vi "Photobleach.vi"(8 "error in (no error)":errorcluster, 10 "Custom Length":dbl=-9999.0, 11 "Stage Controller in":refnum<class "Stage Controller.lvclass">) -> (0 "error out":errorcluster, 3 "Stage Controller out":refnum<class "Stage Controller.lvclass">)   [LabVIEW 2018, in "Stage Controller.lvlib" / "Stage Controller.lvclass"]
uses:
  Stage Controller.lvclass
  Stage Controller.lvclass/Stage Controller.ctl
  <instrlib>/ASI TG-1000/Public/Utility/Axis Name.ctl
  Resources/GLOBAL/GLOBAL Time-critical.vi
  Ti2/ti2lv/ti2lv.lvlib
  <instrlib>/ASI TG-1000/ASI TG-1000.lvlib
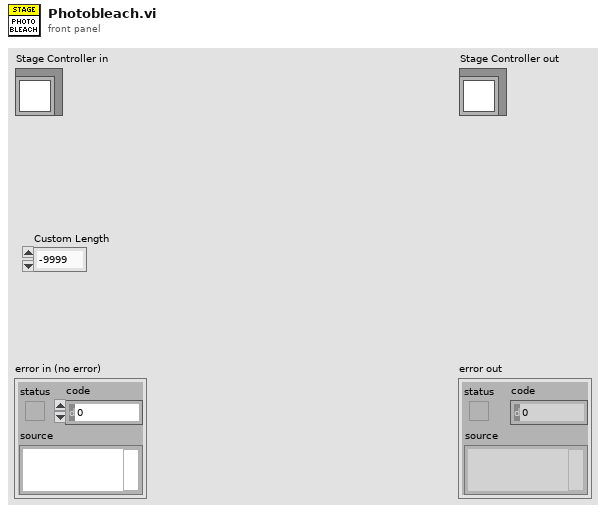
[diagram p1: front panel]
types:
  T1 = enum16{"Disabled", "ESP301", "Ti2", "Ludl", "ASI"}
  T2 = typedef "ASI TG-1000.lvlib/Axis Name.ctl" = enum8{"undefined", "A", "B", "C", "D", "E", "F", "G", "H", "I", "J", "K", "L", "M", "N", "O", "P", "Q", "R", "S", "T", "U", "V", "W", "X", "Y", "Z"}
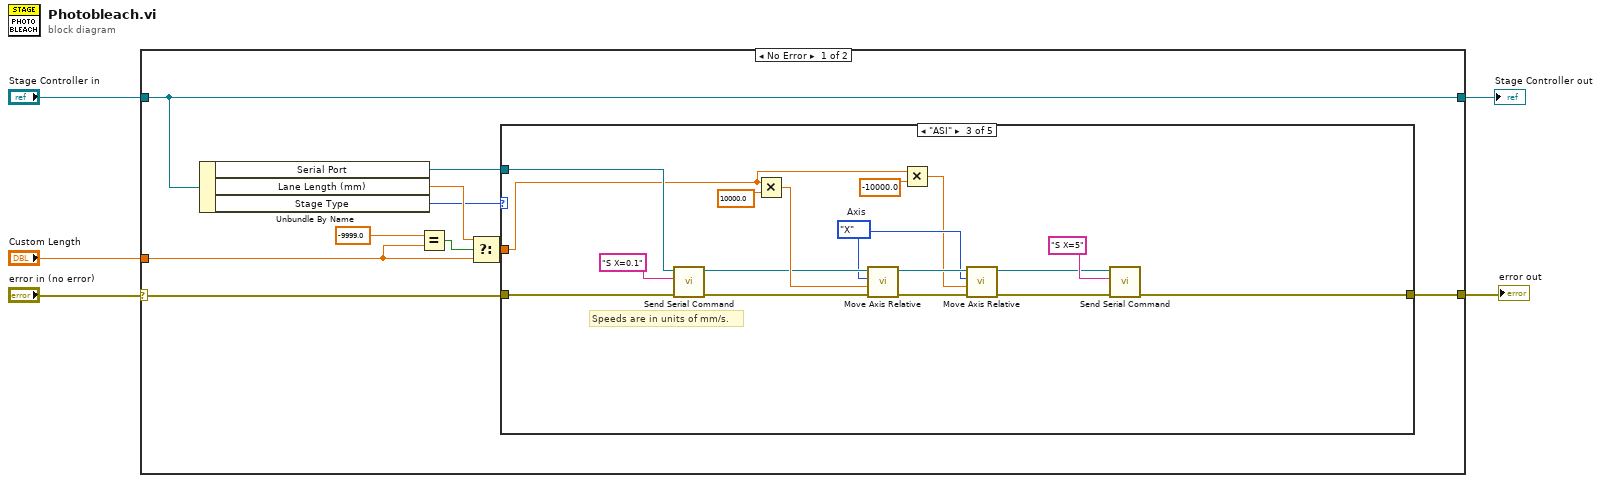
[diagram p0: block diagram]
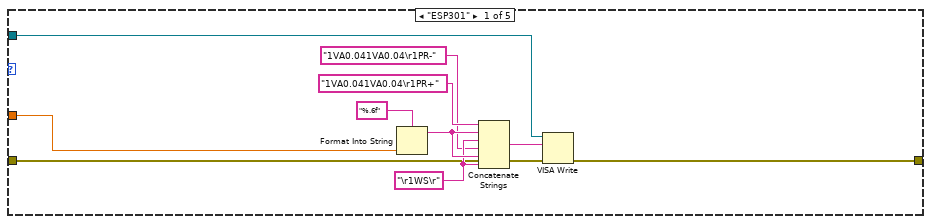
[diagram p2: hidden frame]
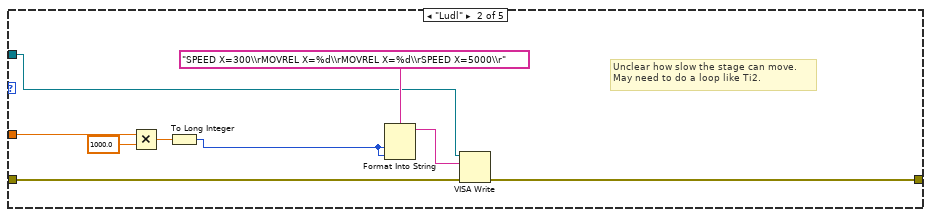
[diagram p3: hidden frame]
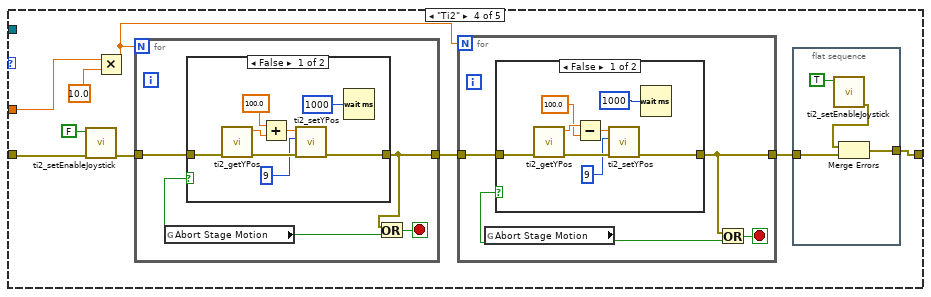
[diagram p4: hidden frame]
diagram:
  n1 = case shown="No Error" "error in (no error)" {
    selector: "error in (no error)" -> [w14 w93]
    tunnel: [w13 w93] -> w4
    tunnel: [w15 w92] -> w2
    tunnel: "Stage Controller in" -> [w15 w92]
    tunnel: "Custom Length" -> [w8 _]
    frame No Error {
      n2 = Unbundle By Name(w15) -> ("Serial Port"=w12:refnum<visa-resource-name>, "Lane Length (mm)"=w10:dbl, "Stage Type"=w6:T1)
      n3 = Equal?(x=-9999.0, y=w8) -> (x = y?=w9:bool)
      n4 = Select(t=w10, s=w9, f=w8) -> (s? t:f=w11:dbl)
      n5 = case shown="\"ASI\"" w6 {
        tunnel: w14 -> [w18 w30 w49 w56 w91]
        tunnel: w11 -> [w17 w33 w35 w59 _]
        tunnel: [w19 w27 w45 w54 w91] -> w13
        tunnel: w12 -> [w16 w28 w44 _ _]
        frame "ESP301" {
          w21 = "\r1WS\r" ("write buffer")
          n6 = Format Into String(format string="%.6f", w17) -> (resulting string=w25:string)  [unwired: 2 in, 1 out]
          n7 = Concatenate Strings("1VA0.041VA0.04\r1PR+" ("write buffer"), w25, w21, "1VA0.041VA0.04\r1PR-" ("write buffer"), w25, w21) -> (w24:string)
          n8 = VISA Write(VISA resource name=w16, write buffer=w24, error in (no error)=w18) -> (error out=w19:errorcluster)  [unwired: 2 out]
        }
        frame "Ludl" {
          # "Unclear how slow the stage can move.\nMay need to do a loop like Ti2."
          n9 = Multiply(x=w33, y=1000.0) -> (x*y=w31:dbl)
          n10 = To Long Integer(number=w31) -> (32bit integer=w26:i32)
          n11 = Format Into String(format string="SPEED X=300\\rMOVREL X=%d\\rMOVREL X=%d\\rSPEED X=5000\\r", w26, w26) -> (resulting string=w34:string)  [unwired: 2 in, 1 out]
          n12 = VISA Write(VISA resource name=w28, write buffer=w34, error in (no error)=w30) -> (error out=w27:errorcluster)  [unwired: 2 out]
        }
        frame "ASI" {
          w38 = Axis_Name."X"  # Axis
          # "Speeds are in units of mm/s."
          n13 = call <instrlib>:"Send Serial Command.vi"("error in (no error)"=w49, "Command"="S X=0.1", "VISA in"=w44) -> ("error out"=w48:errorcluster, "VISA out"=w39:refnum<visa-resource-name>)  [unwired: 6 in, 1 out]
          n14 = Multiply(x=w35, y=10000.0) -> (x*y=w51:dbl)
          n15 = call <instrlib>:"Move Axis Relative.vi"("error in (no error)"=w48, "Relative Position [internal units]"=w51, "Axis"=w38, "VISA in"=w39) -> ("error out"=w43:errorcluster, "VISA out"=w41:refnum<visa-resource-name>)  [unwired: 5 in]
          n16 = Multiply(x=w35, y=-10000.0) -> (x*y=w36:dbl)
          n17 = call <instrlib>:"Move Axis Relative.vi"("error in (no error)"=w43, "Relative Position [internal units]"=w36, "Axis"=w38, "VISA in"=w41) -> ("error out"=w42:errorcluster, "VISA out"=w40:refnum<visa-resource-name>)  [unwired: 5 in]
          n18 = call <instrlib>:"Send Serial Command.vi"("error in (no error)"=w42, "Command"="S X=5", "VISA in"=w40) -> ("error out"=w45:errorcluster)  [unwired: 6 in, 2 out]
        }
        frame "Ti2" {
          n19 = call "ti2_setEnableJoystick.vi"("error in (no error)"=w56, "value"=FALSE) -> ("error out"=w57:errorcluster)  [unwired: 9 in]
          n20 = Multiply(x=w59, y=10.0) -> (x*y=w58:dbl)
          n21 = for {
            N: w58 -> [_]
            tunnel: w57 -> [w81]
            tunnel: [w79] -> w52
            stop <- w80 stop-if-true
            n22 = global read "GLOBAL Time-critical.vi" "Abort Stage Motion"() -> (w78:bool)
            n23 = case shown="False" w78 {
              tunnel: [w83 w90] -> w79
              tunnel: w81 -> [w82 w90]
              frame False {
                n24 = call "ti2_getYPos.vi"("error in (no error)"=w82) -> ("error out"=w89:errorcluster, "y Position (um)"=w87:dbl)  [unwired: 9 in]
                n25 = Add(x=100.0, y=w87) -> (x+y=w88:dbl)
                n26 = call "ti2_setYPos.vi"("error in (no error)"=w89, "speed"=9, "y Position (um)"=w88) -> ("error out"=w83:errorcluster)  [unwired: 8 in]
                n27 = Wait (ms)(milliseconds to wait=u32 1000) -> ()  [unwired: 1 out]
              }
              frame True {
              }
            }
            n28 = Or(x=w79, y=w78) -> (x .or. y?=w80:bool)
          }
          n29 = for {
            N: w58 -> [_]
            tunnel: w52 -> [w64]
            tunnel: [w62] -> w53
            stop <- w63 stop-if-true
            n30 = global read "GLOBAL Time-critical.vi" "Abort Stage Motion"() -> (w61:bool)
            n31 = case shown="False" w61 {
              tunnel: [w66 w73] -> w62
              tunnel: w64 -> [w65 w73]
              frame False {
                n32 = call "ti2_getYPos.vi"("error in (no error)"=w65) -> ("error out"=w72:errorcluster, "y Position (um)"=w70:dbl)  [unwired: 9 in]
                n33 = Subtract(x=w70, y=100.0) -> (x-y=w71:dbl)
                n34 = call "ti2_setYPos.vi"("error in (no error)"=w72, "speed"=9, "y Position (um)"=w71) -> ("error out"=w66:errorcluster)  [unwired: 8 in]
                n35 = Wait (ms)(milliseconds to wait=u32 1000) -> ()  [unwired: 1 out]
              }
              frame True {
              }
            }
            n36 = Or(x=w62, y=w61) -> (x .or. y?=w63:bool)
          }
          n37 = flat-sequence {
            tunnel: [w76] -> w54
            tunnel: w53 -> [w74]
            frame #0 {
              n38 = call "ti2_setEnableJoystick.vi"("value"=TRUE) -> ("error out"=w75:errorcluster)  [unwired: 10 in]
              n39 = Merge Errors(w75, w74) -> (w76:errorcluster)
            }
          }
        }
        frame "Disabled", Default {
        }
      }
    }
    frame Error {
    }
  }
  "error out" <- w4
  "Stage Controller out" <- w2
